vi "ToggleContinousMode_.vi"(8 "error in":errorcluster, 10 "Cont Acquisition":bool, 11 "scope in":T1) -> (0 "error out":errorcluster, 3 "scope out":T1)   [LabVIEW 2013]
uses:
  Scope/controls/AcquisitionTriggerFPGARef.ctl
  <vilib>/rvi/interface/common/niFpgaWaitOnOcc.vi
  <vilib>/Utility/error.llb/Error Cluster From Error Code.vi
  <vilib>/rvi/errors/niLvFpgaAdjustHostInterfaceError.vi
  <vilib>/rvi/interface/nirviReadWriteControl/nirviReadWriteControl.xnode
  NiFpgaLv.dll
  <vilib>/rvi/interface/Simulation/niFpgaSimulationCallBeginRW.vi
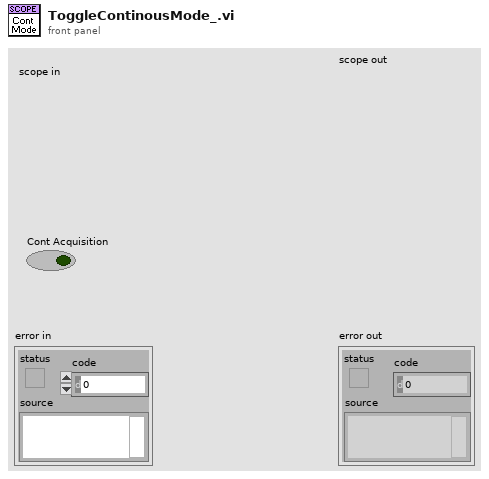
[diagram p1: front panel]
types:
  T1 = typedef "AcquisitionTriggerFPGARef.ctl" = refnum<k20>
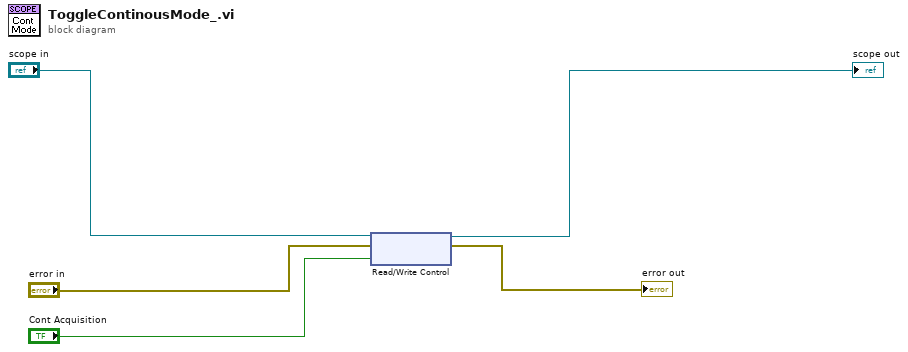
[diagram p0: block diagram]
diagram:
  n1 = xnode "Read/Write Control"("FPGA VI Reference In"="scope in", "error in"="error in", "Continuous"="Cont Acquisition") -> ("FPGA VI Reference Out"=→"scope out":T1, "error out"=→"error out":errorcluster)
